vi "Process.vi"(8 "error in":errorcluster, 11 "Log.Litho":refnum<class "Log.Litho.lvclass">) -> (0 "error out":errorcluster, 3 "Log.Litho out":refnum<class "Log.Litho.lvclass">)   [LabVIEW 2019, in "Log.Litho.lvclass"]
doc: "---------------------------------------------------------------\nJKI State Machine Objects™\nhttp://jki.net/state-machine-objects/\nCopyright (C) 2005-2015, JKI <info@jki.net>\nALL RIGHTS RESERVED"
uses:
  Log.Litho.lvclass
  C:/Program Files (x86)/National Instruments/LabVIEW 2019/vi.lib/JKI/JKI SMO/SMO/SMO.lvclass
  <vilib>/JKI/JKI SMO/SMO/Typedefs/Parent Call--Enum.ctl
  <vilib>/JKI/JKI SMO/SMO/SMO.lvclass/SMO.ctl
  Log.Litho.lvclass/Log.Litho.ctl
  <vilib>/JKI/JKI SMO/SMO/Private/ReftoDVR--SMO.vi
  <vilib>/JKI/JKI SMO/SMO/SMO.lvclass
panel:
  # "For instructions on how to use the JKI State Machine Objects, examples and video tutorials, visit:\nhttp://jki.net/state-machine-objects/\n\nJKI State Machine Objects™\nhttp://jki.net/state-machine-objects/\nCopyright (C) 2005-2015, JKI <info@jki.net>\nALL RIGHTS RESERVED"
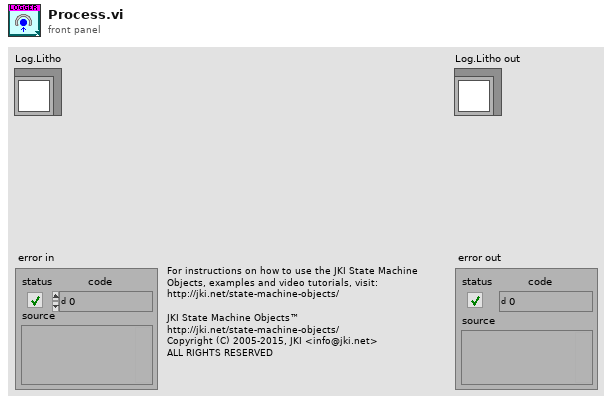
[diagram p1: front panel]
types:
  T1 = typedef "SMO.lvclass/Parent Call--Enum.ctl" = enum16{"Allows parent to run", "Does not request parent to run"}
  T2 = enum32{"invalid app kind", "Development System", "Run Time System", "Student Edition", "Embedded LabVIEW", "Evaluation", "Custom"}
  T3 = enum32{"Invalid", "Standard", "Closed", "Hidden", "Minimized", "Maximized"}
  T4 = enum32{"Bad", "Idle", "Run top level", "Running"}
  T5 = enum16{"open", "replace", "create", "open or create", "replace or create", "replace or create with confirmation"}
  T6 = typedef "Log.Litho.lvclass/PrivateEvents--Log.Litho.Activity.ctl" = string
  T7 = cluster{"Core":cluster{"Current VI Reference":refnum<vi>, "Close Panel on Exit?":bool, "error":errorcluster}, "Self Reference":refnum<class "Log.Litho.lvclass">, "Activity":string, "Path":path, "Active Log":string, "File Refnum":refnum<file>}
  T8 = cluster{"Current VI Reference":refnum<vi>, "Close Panel on Exit?":bool, "error":errorcluster}
  T9 = typedef "SMO.lvclass/Protected Events.ctl" = cluster{"StopProcesses":refnum<user-event>, "AbortProcesses":refnum<user-event>, "Config Changed":refnum<user-event>, "Dependency":refnum<user-event>}
  T10 = typedef "Log.Litho.lvclass/PrivateEvents--Cluster.ctl" = cluster{"Activity":refnum<user-event>}
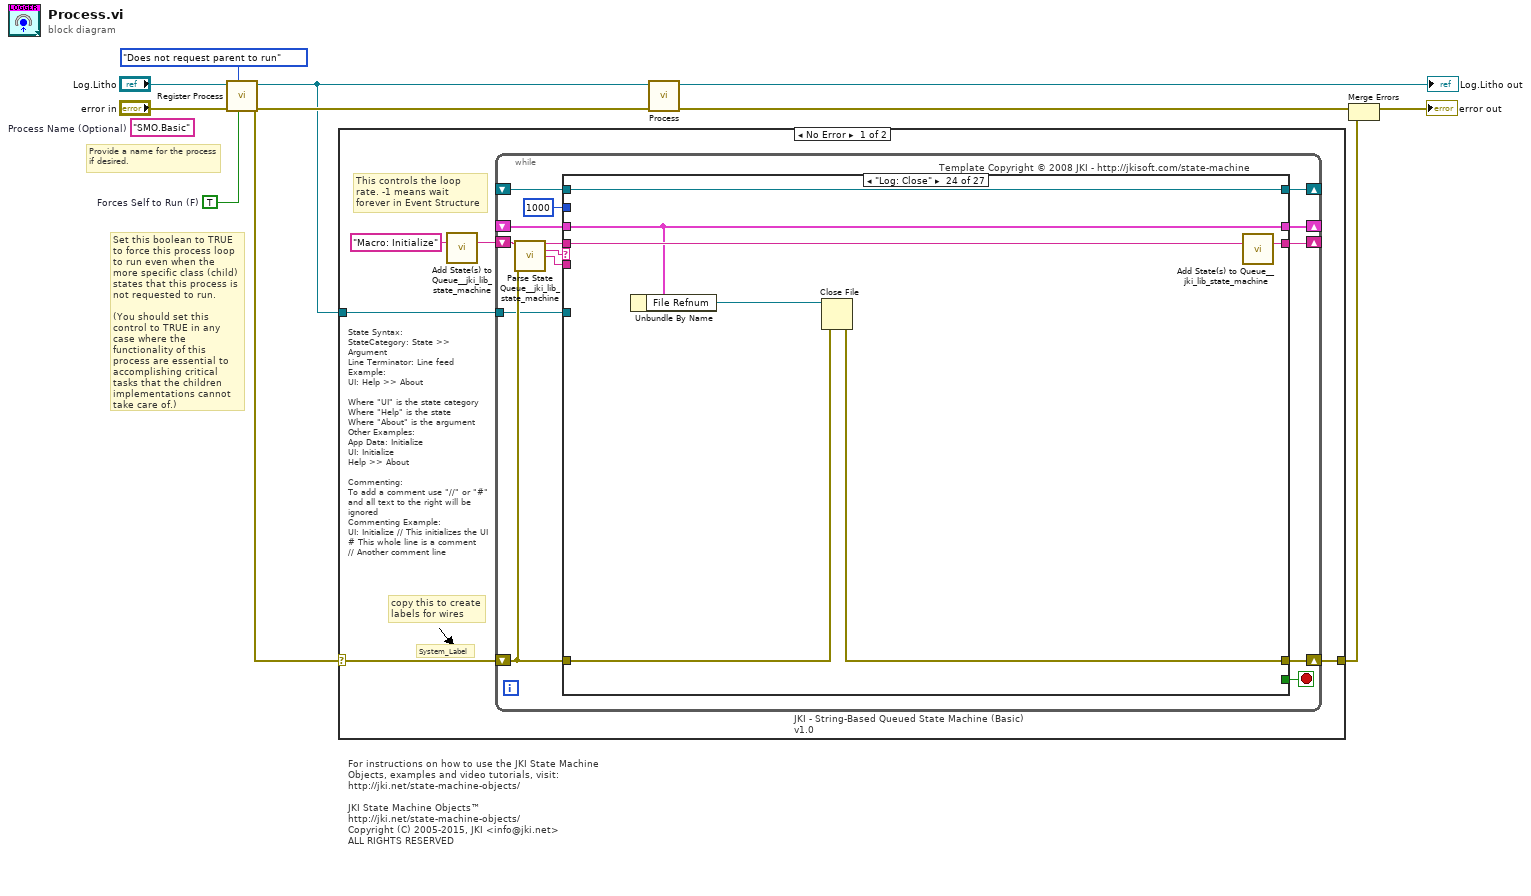
[diagram p0: block diagram]
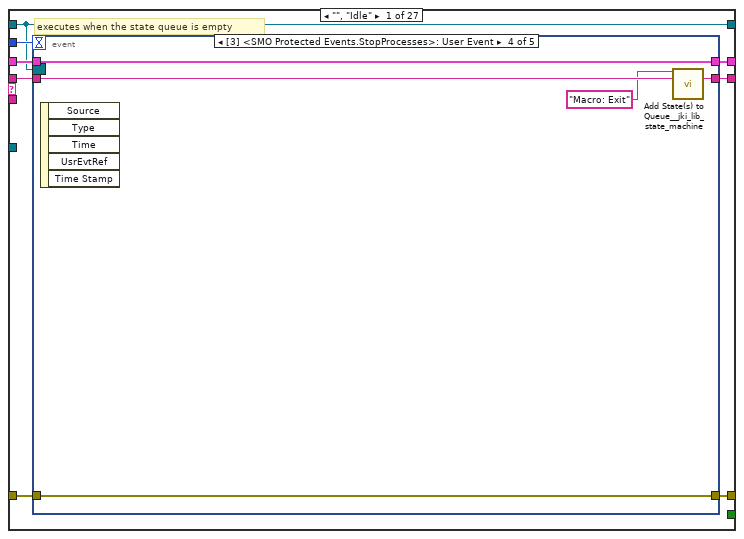
[diagram p2: hidden frame]
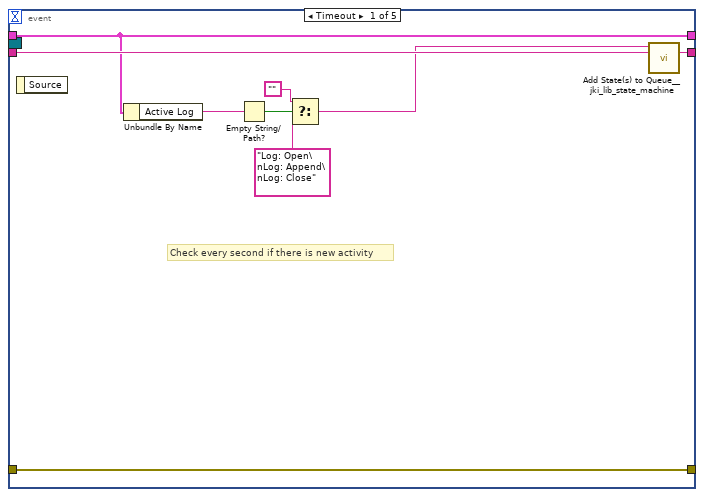
[diagram p3: hidden frame]
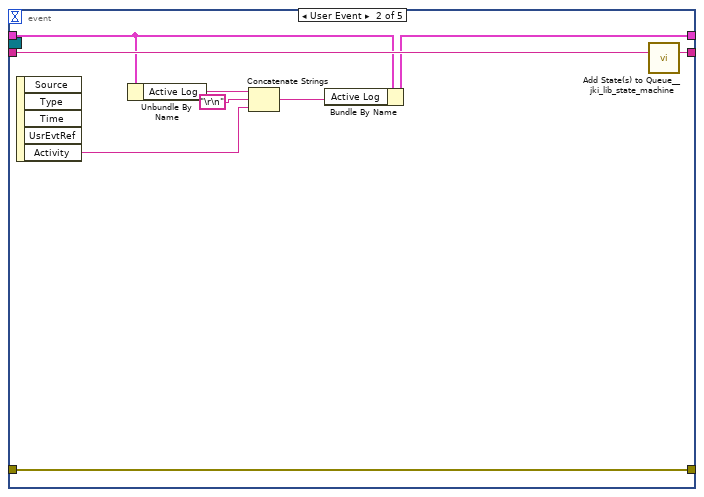
[diagram p4: hidden frame]
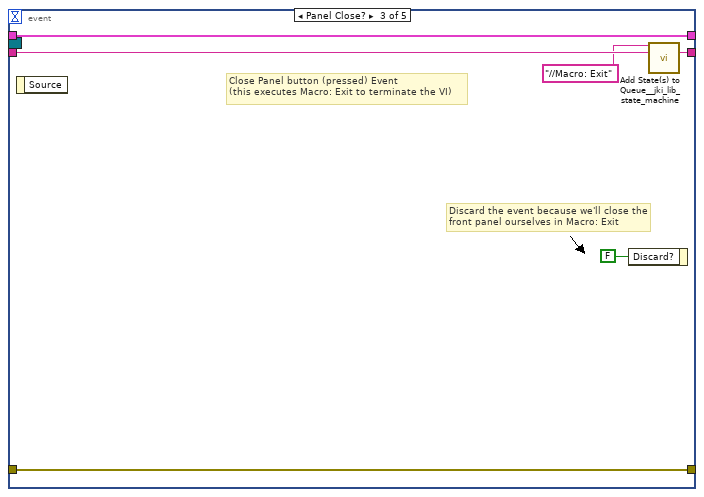
[diagram p5: hidden frame]
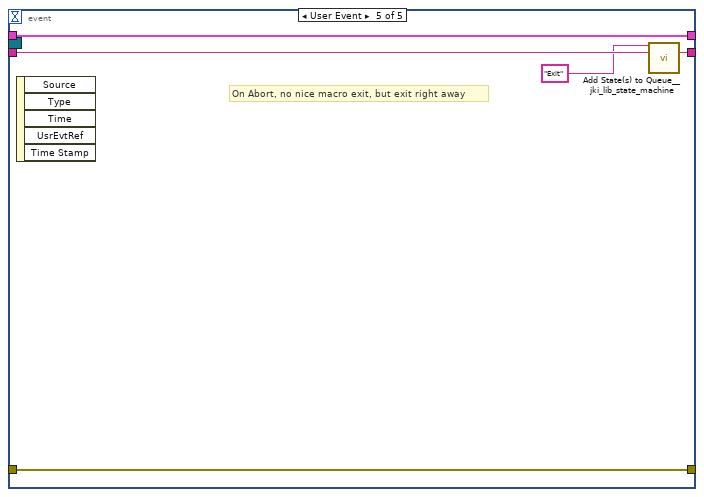
[diagram p6: hidden frame]
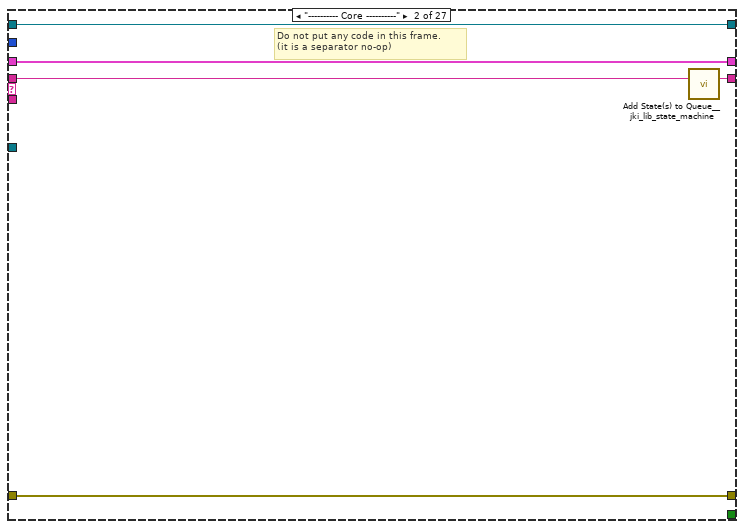
[diagram p7: hidden frame]
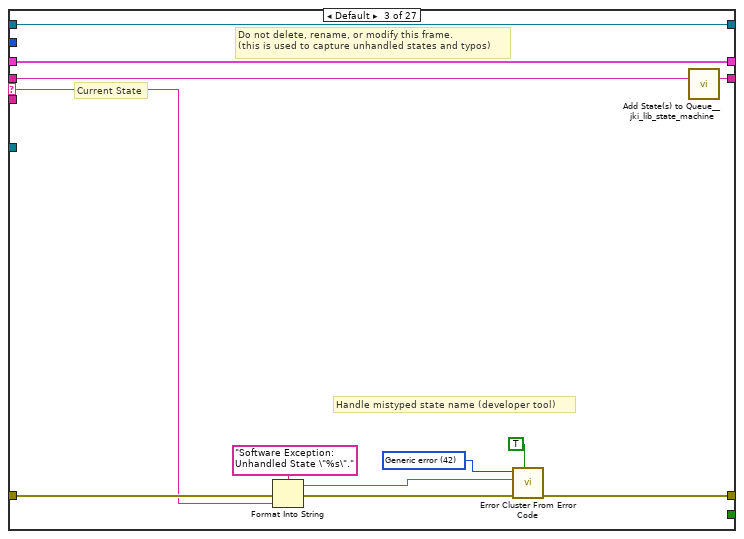
[diagram p8: hidden frame]
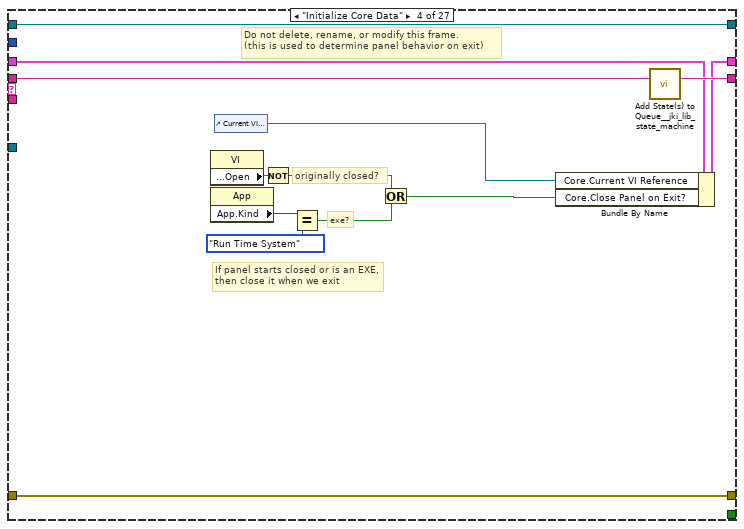
[diagram p9: hidden frame]
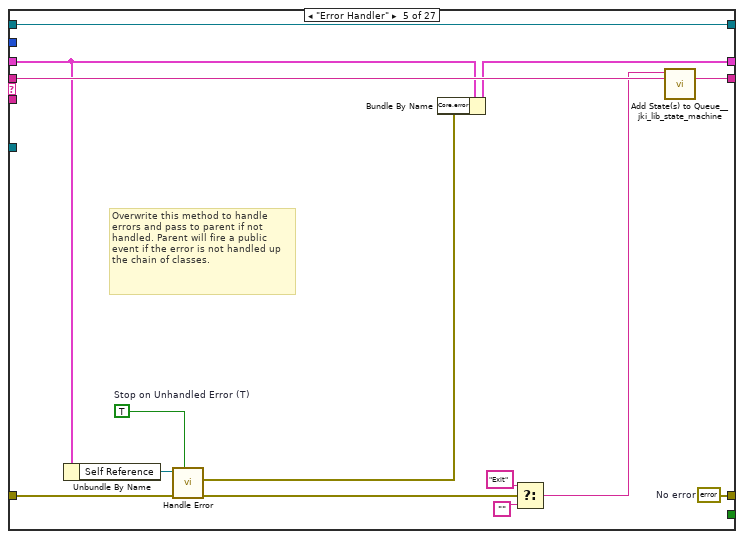
[diagram p10: hidden frame]
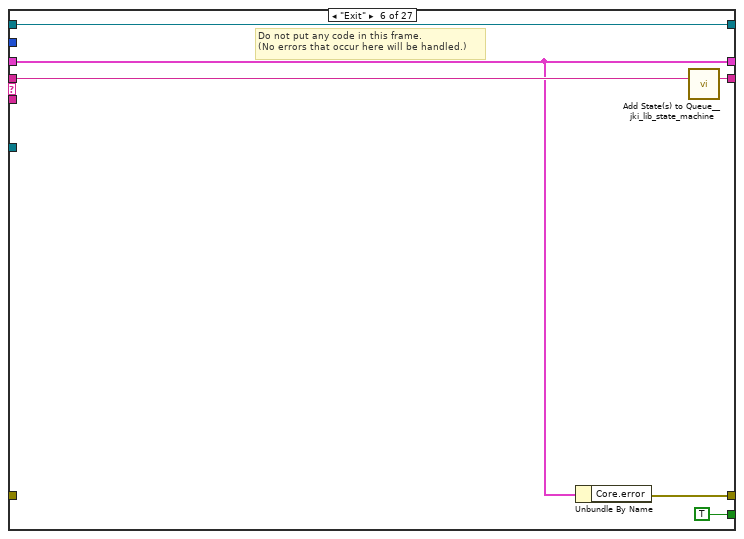
[diagram p11: hidden frame]
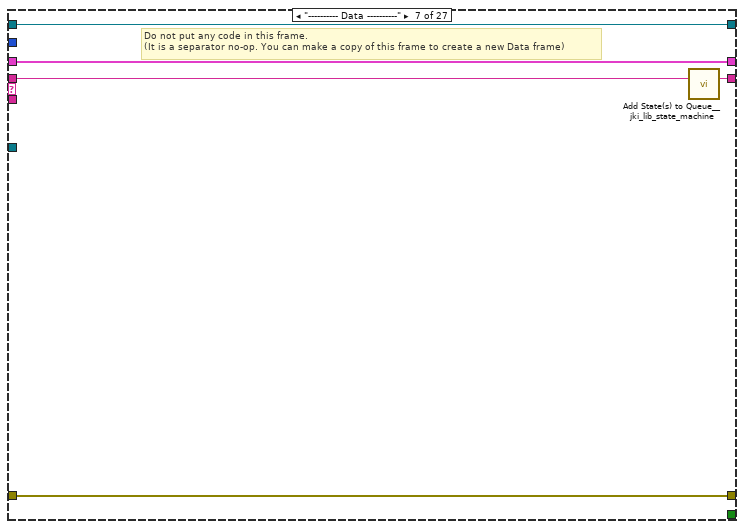
[diagram p12: hidden frame]
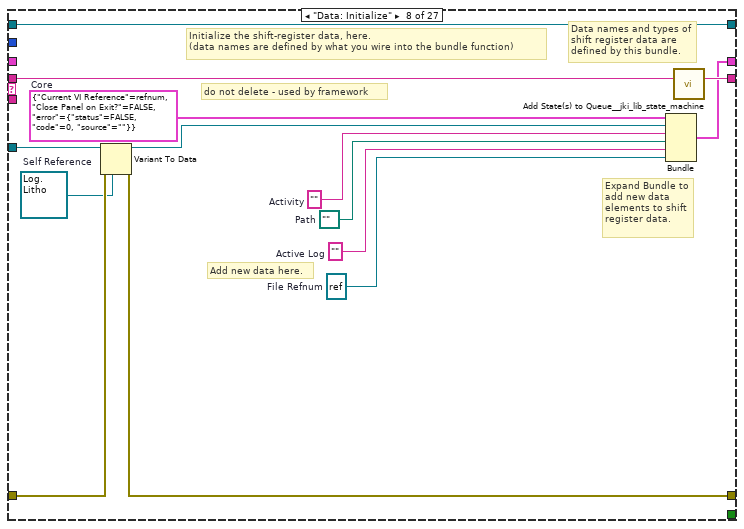
[diagram p13: hidden frame]
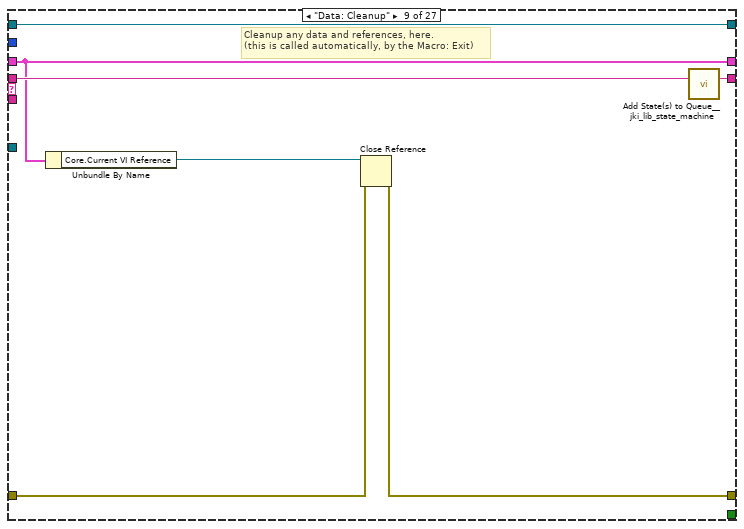
[diagram p14: hidden frame]
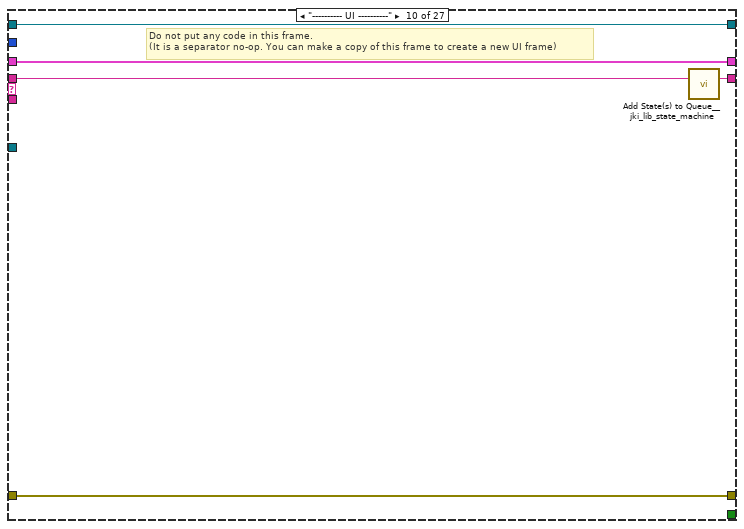
[diagram p15: hidden frame]
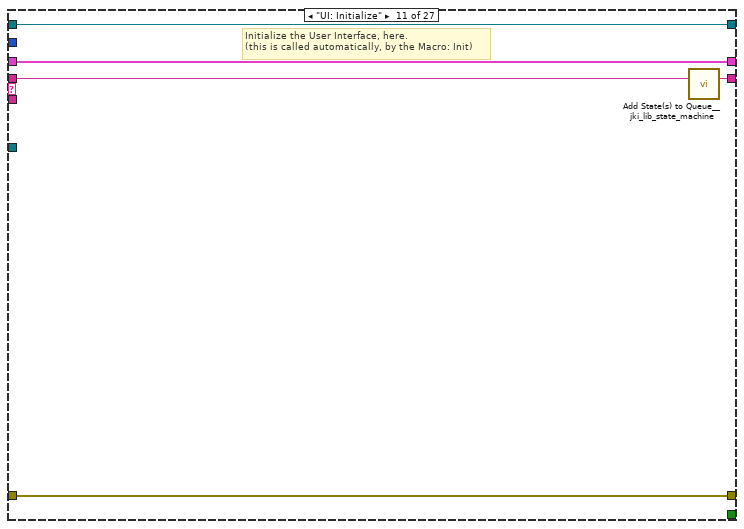
[diagram p16: hidden frame]
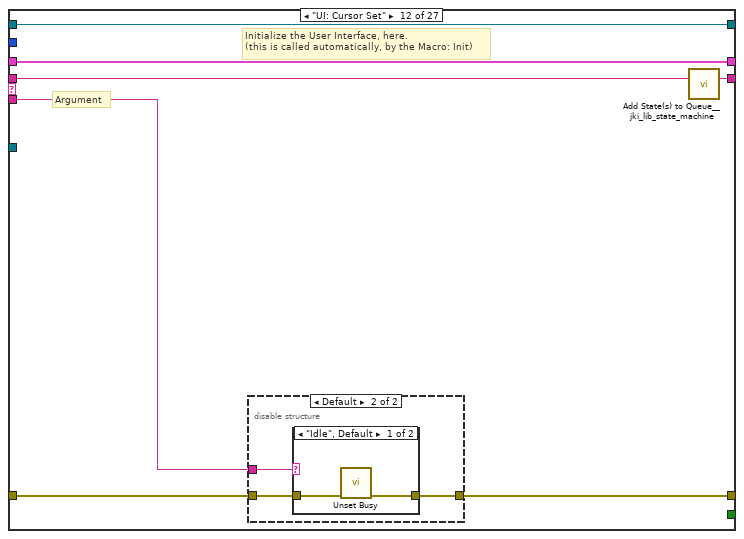
[diagram p17: hidden frame]
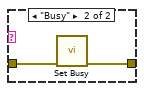
[diagram p19: hidden frame]
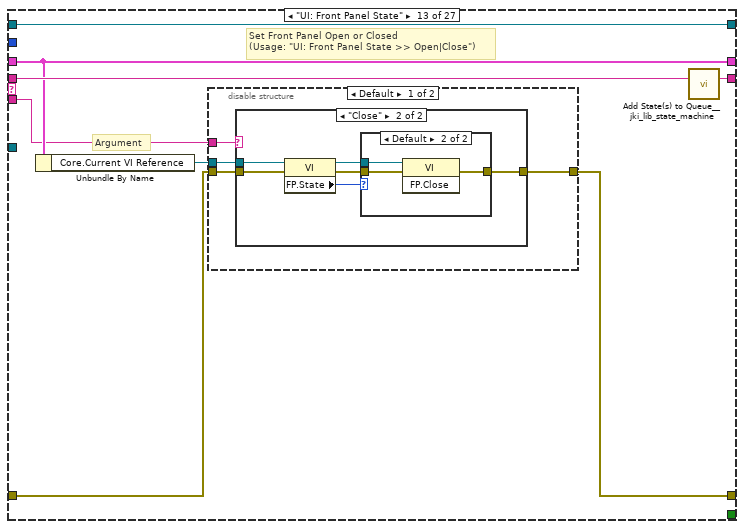
[diagram p20: hidden frame]
diagram:
  w1 = TRUE  # Forces Self to Run (F)
  (unwired) "SMO.Basic"  # Process Name (Optional)
  # "Provide a name for the process\nif desired."
  # "Set this boolean to TRUE to force this process loop to run even when the more specific class (child) states that this process is not requested to run.\n\n(You should set this control to TRUE in any case where the functionality of this process are essential to accomplishing critical tasks that the children implementations cannot take care of.)"
  # "For instructions on how to use the JKI State Machine Objects, examples and video tutorials, visit:\nhttp://jki.net/state-machine-objects/\n\nJKI State Machine Objects™\nhttp://jki.net/state-machine-objects/\nCopyright (C) 2005-2015, JKI <info@jki.net>\nALL RIGHTS RESERVED"
  n1 = call <vilib>:"Register Process.vi"("Forces Self to Run (F)"=w1, "Parent Call"=Parent_Call--Enum."Does not request parent to run", "error in (no error)"="error in", "SMO"="Log.Litho") -> ("error out"=w7:errorcluster, "SMO out"=w6:refnum<class "Log.Litho.lvclass">)  [unwired: 6 in]
  n2 = case shown="No Error" w7 {
    selector: w7 -> [w12 w342]
    tunnel: w6 -> [w13 _]
    tunnel: [w11 w342] -> w3
    frame No Error {
      # "State Syntax:\nStateCategory: State >> Argument\nLine Terminator: Line feed\nExample:\nUI: Help >> About\n\nWhere \"UI\" is the state category\nWhere \"Help\" is the state\nWhere \"About\" is the argument\nOther Examples:\nApp Data: Initialize\nUI: Initialize\nHelp >> About\n\nCommenting:\nTo add a comment use \"//\" or \"#\" and all text to the right will be ignored\nCommenting Example:\nUI: Initialize // This initializes the UI\n# This whole line is a comment\n// Another comment line"
      # "copy this to create labels for wires"
      # "This controls the loop rate. -1 means wait forever in Event Structure"
      # "System_Label"
      n3 = call <vilib>:"Add State(s) to Queue__jki_lib_state_machine.vi"("State(s) in (\"\")"="Macro: Initialize") -> ("States Out"=w15:string)  [unwired: 14 in]
      n4 = while "JKI - String-Based Queued State Machine (Basic) v1.0" {
        shift-right: [w22] -> _
        shift-left: _ -> [w21]
        shift-right: [w25] -> w11
        shift-left: w12 -> [w19]
        shift-right: [w24] -> _
        shift-left: w15 -> [w26]
        tunnel: w13 -> [w18]
        shift-right: [w17] -> _
        shift-left: _ -> [w16]
        stop <- w23 stop-if-true
        # "Template Copyright © 2008 JKI - http://jkisoft.com/state-machine"
        n5 = call <vilib>:"Parse State Queue__jki_lib_state_machine.vi"("State Queue"=w26, "Error In (no error)"=w19) -> ("Remaining States"=w28:string, "Current State"=w29:string, "Arguments"=w27:string)  [unwired: 11 in]
        n6 = case shown="\"Log: Close\"" w29 {
          selector: w29 -> [_ _ w78 _ _ _ _ _ _ _ _ _ _ _ _ _ _ _ _ _ _ _ _ _ _ _ _]
          tunnel: w28 -> [w37 w76 w82 w101 w115 w121 w126 w140 w147 w152 w157 w164 w180 w212 w226 w240 w245 w256 w261 w273 w279 w284 w300 w307 w317 w333 w341]
          tunnel: w27 -> [_ _ _ _ _ _ _ _ _ _ _ w158 w174 _ _ _ _ _ _ _ _ _ _ _ _ _ _]
          tunnel: w21 -> [w35 w73 w80 w92 w109 w117 w123 _ w142 w149 w155 w162 w176 w209 w222 w231 w242 w253 w258 w271 w277 w282 w288 w304 w308 w320 w334]
          tunnel: [w34 w74 w84 w98 w110 w116 w124 w135 w143 w150 w154 w159 w177 w210 w224 w238 w243 w247 w259 w267 w275 w280 w291 w302 w312 w323 w337] -> w25
          tunnel: w19 -> [w33 w74 w83 w98 w111 _ w124 w136 w144 w150 w154 w160 w178 w210 w224 w238 w243 w248 w259 w268 w275 w280 w290 w301 w311 w322 w338]
          tunnel: [w36 w75 w81 w100 w114 w120 w125 w139 w146 w151 w156 w163 w179 w211 w225 w239 w244 w255 w260 w272 w278 w283 w299 w306 w316 w332 w340] -> w24
          tunnel: [_ _ _ _ _ TRUE _ _ _ _ _ _ _ _ _ _ _ _ _ _ _ _ _ _ _ _ _] -> w23
          tunnel: [w32 w73 w80 w99 w108 w117 w123 w138 w142 w149 w155 w162 w176 w209 w222 w231 w242 w253 w258 w271 w277 w282 w289 w304 w309 w321 w335] -> w22
          tunnel: 1000 ("Timeout") -> [w31 _ _ _ _ _ _ _ _ _ _ _ _ _ _ _ _ _ _ _ _ _ _ _ _ _ _]
          tunnel: w18 -> [_ _ _ _ _ _ _ w133 _ _ _ _ _ _ _ _ _ _ _ _ _ _ _ _ _ _ _]
          tunnel: [w30 w72 w77 w89 w113 w118 w122 w131 w141 w148 w153 w161 w173 w208 w223 w232 w241 w254 w257 w270 w276 w281 w298 w305 w315 w331 w339] -> w17
          tunnel: w16 -> [w30 w72 w77 w89 w113 w118 w122 w131 w141 w148 w153 w161 w173 w208 w223 w232 w241 w254 w257 _ w276 w281 w298 w305 w315 w331 w339]
          frame "", "Idle" {
            # "executes when the state queue is empty"
            n7 = event shown="[3] <SMO Protected Events.StopProcesses>: User Event" {
              selector: w30 -> [_ _ _ _ _]
              dyn-events: _ -> [_ _ _ _ _]
              timeout: w31 -> [_ _ _ _ _]
              tunnel: w37 -> [w46 w55 w61 w66 w71]
              tunnel: [w45 w54 w60 w65 w70] -> w36
              tunnel: w35 -> [w43 w49 w58 w63 w68]
              tunnel: [w44 w53 w59 w64 w69] -> w34
              tunnel: w33 -> [w44 w53 w59 w64 w69]
              tunnel: [w43 w50 w58 w63 w68] -> w32
              event Timeout {
                # "Check every second if there is new activity"
                n8 = event-data() -> ()  [unwired: 1 in, 1 out]
                n9 = Unbundle By Name(w43) -> ("Active Log"=w42:string)
                n10 = Empty String/Path?(string/path=w42) -> (empty?=w41:bool)
                n11 = Select(t="", s=w41, f="Log: Open\nLog: Append\nLog: Close") -> (s? t:f=w38:string)
                n12 = call <vilib>:"Add State(s) to Queue__jki_lib_state_machine.vi"("State(s) in Front (\"\")"=w38, "State(s) in (\"\")"=w46) -> ("States Out"=w45:string)  [unwired: 13 in]
              }
              event User Event {
                n13 = event-data() -> ("Activity"=w48:T6)  [unwired: 1 in, 4 out]
                n14 = Unbundle By Name(w49) -> ("Active Log"=w52:string)
                n15 = Concatenate Strings(w52, "\r\n", w48) -> (w47:string)
                n16 = Bundle By Name(cluster=w49, "Active Log"=w47) -> (w50:T7)
                n17 = call <vilib>:"Add State(s) to Queue__jki_lib_state_machine.vi"("State(s) in (\"\")"=w55) -> ("States Out"=w54:string)  [unwired: 14 in]
              }
              event Panel Close? {
                # "Discard the event because we'll close the front panel ourselves in Macro: Exit"
                # "Close Panel button (pressed) Event\n(this executes Macro: Exit to terminate the VI)"
                n18 = event-data() -> ()  [unwired: 1 in, 1 out]
                n19 = event-data("Discard?"=FALSE) -> ()  [unwired: 1 in, 1 out]
                n20 = call <vilib>:"Add State(s) to Queue__jki_lib_state_machine.vi"("State(s) in Front (\"\")"="//Macro: Exit", "State(s) in (\"\")"=w61) -> ("States Out"=w60:string)  [unwired: 13 in]
              }
              event User Event {
                n21 = event-data() -> ()  [unwired: 1 in, 5 out]
                n22 = call <vilib>:"Add State(s) to Queue__jki_lib_state_machine.vi"("State(s) in Front (\"\")"="Macro: Exit", "State(s) in (\"\")"=w66) -> ("States Out"=w65:string)  [unwired: 13 in]
              }
              event User Event {
                # "On Abort, no nice macro exit, but exit right away"
                n23 = event-data() -> ()  [unwired: 1 in, 5 out]
                n24 = call <vilib>:"Add State(s) to Queue__jki_lib_state_machine.vi"("State(s) in Front (\"\")"="Exit", "State(s) in (\"\")"=w71) -> ("States Out"=w70:string)  [unwired: 13 in]
              }
            }
          }
          frame "---------- Core ----------" {
            # "Do not put any code in this frame.\n(it is a separator no-op)"
            n25 = call <vilib>:"Add State(s) to Queue__jki_lib_state_machine.vi"("State(s) in (\"\")"=w76) -> ("States Out"=w75:string)  [unwired: 14 in]
          }
          frame Default {
            w87 = 42 items=["No error", "Argument error", "Memory is full", "Out of zone", "End of file", "File already open", "Generic file I/O error", "File not found", "File permission error", "Disk is full", "Duplicate path", "Too many files open", "System feature not enabled", "Resource file not found", "Cannot add resource", "Resource not found", "Image not found", "Image memory error", "Pen does not exist", "Config type invalid", "Config token not found", "Config parse error", "Config memory error", "Bad external code format", "Bad external code offset", "External code not present", "Null window", "Destroy window error", "Null menu", "Print aborted", "Bad print record", "Print driver error", "Windows error during printing", "Memory error during printing", "Print dialog error", "Generic print error", "Invalid device refnum", "Device not found", "Device parameter error", "Device unit error", "Cannot open device", "Device call aborted", "Generic error", "Cancelled by user", "Object ID too low", "Object ID too high", "Object not in heap", "Unknown heap", "Unknown object (invalid DefProc)", "Unknown object (DefProc not in table)", "Message out of range", "Invalid (null) method", "Unknown message", "Manager call not supported", "Bad address", "Network operation in progress", "Network operation timed out", "Connection is busy", "Network attribute not supported", "Network error", "Address in use", "System out of memory", "Connection aborted", "Connection refused", "Not connected", "Already connected", "Connection closed", "Initialization error (interapplication manager)", "Bad occurrence", "Wait on unbound occurrence handler", "Occurrence queue overflow", "Datalog type conflict", "Unused", "Unrecognized type (interapplication manager)", "Memory corrupt", "Failed to make temporary DLL", "Old CIN version", "Drag socket not found", "Failed to load drop-object", "Failed to register OLE object", "Failed to release OLE object", "Format specifier type mismatch", "Unknown format specifier", "Too few format specifiers", "Too many format specifiers", "Scan failed", "Newer CIN version", "Error converting to variant", "Runtime menu error", "Password tampered", "Variant attribute not found", "Incompatible variant data type", "Event data is not available", "Event Store is not present", "Occurrence is not found", "Event Queue is not created", "Event info is not available", "Refnum passed is NULL", "Error retrieving Class GUID", "Error retrieving CoClass GUID", "Error retrieving TypeLib GUID.", "Bad built application magic bytes.", "Specific driver is different from the specific driver associated with the Logical Name.", "There is no session opened to the class driver.", "Max Error", "MAX - Error with config objects", "MAX - Error loading configuration", "MAX - Group not supported"]
            # "Current State"
            # "Do not delete, rename, or modify this frame.\n(this is used to capture unhandled states and typos)"
            # "Handle mistyped state name (developer tool)"
            n26 = Format Into String(format string="Software Exception: Unhandled State \"%s\"." ("message"), error in=w83, w78) -> (resulting string=w86:string, error out=w85:errorcluster)  [unwired: 1 in]
            n27 = call <vilib>:"Error Cluster From Error Code.vi"("show call chain? (False)"=TRUE, "error in (no error)"=w85, "error message (\"\")"=w86, "error code (0)"=w87) -> ("error out"=w84:errorcluster)  [unwired: 5 in]
            n28 = call <vilib>:"Add State(s) to Queue__jki_lib_state_machine.vi"("State(s) in (\"\")"=w82) -> ("States Out"=w81:string)  [unwired: 14 in]
          }
          frame "Initialize Core Data" {
            # "Do not delete, rename, or modify this frame.\n(this is used to determine panel behavior on exit)"
            # "originally closed?"
            # "exe?"
            # "If panel starts closed or is an EXE, then close it when we exit"
            n29 = property class="VI"() -> ("Front Panel.Open"=w97:bool)  [unwired: 2 in, 2 out]
            n30 = property class="App"() -> ("App.Kind"=w96:T2)  [unwired: 2 in, 2 out]
            n31 = control-ref of="Current VI Reference"() -> (w90:refnum<vi>)
            n32 = Not(x=w97) -> (.not. x?=w94:bool)
            n33 = Equal?(x=w96, y=T2."Run Time System" ("Application:Kind")) -> (x = y?=w93:bool)
            n34 = Or(x=w94, y=w93) -> (x .or. y?=w91:bool)
            n35 = Bundle By Name(cluster=w92, "Core.Current VI Reference"=w90, "Core.Close Panel on Exit?"=w91) -> (w99:T7)
            n36 = call <vilib>:"Add State(s) to Queue__jki_lib_state_machine.vi"("State(s) in (\"\")"=w101) -> ("States Out"=w100:string)  [unwired: 14 in]
          }
          frame "Error Handler" {
            w102 = TRUE  # Stop on Unhandled Error (T)
            w110 = errorcluster {"status"=FALSE, "code"=0, "source"=""}  # No error
            # "Overwrite this method to handle errors and pass to parent if not handled. Parent will fire a public event if the error is not handled up the chain of classes."
            n37 = Unbundle By Name(w109) -> ("Self Reference"=w112:refnum<class "Log.Litho.lvclass">)
            n38 = call-dynamic "Handle Error.vi"("Stop on Unhandled Error (T)"=w102, "error in"=w111, "SMO"=w112) -> ("handling error"=w103:errorcluster, "Unhandled error"=w106:errorcluster)  [unwired: 6 in, 1 out]
            n39 = Bundle By Name(cluster=w109, "Core.error"=w106) -> (w108:T7)
            n40 = Select(t="Exit", s=w103, f="") -> (s? t:f=w107:string)
            n41 = call <vilib>:"Add State(s) to Queue__jki_lib_state_machine.vi"("State(s) in Front (\"\")"=w107, "State(s) in (\"\")"=w115) -> ("States Out"=w114:string)  [unwired: 13 in]
          }
          frame "Exit" {
            # "Do not put any code in this frame.\n(No errors that occur here will be handled.)"
            n42 = Unbundle By Name(w117) -> ("Core.error"=w116:errorcluster)
            n43 = call <vilib>:"Add State(s) to Queue__jki_lib_state_machine.vi"("State(s) in (\"\")"=w121) -> ("States Out"=w120:string)  [unwired: 14 in]
          }
          frame "---------- Data ----------" {
            # "Do not put any code in this frame.\n(It is a separator no-op. You can make a copy of this frame to create a new Data frame)"
            n44 = call <vilib>:"Add State(s) to Queue__jki_lib_state_machine.vi"("State(s) in (\"\")"=w126) -> ("States Out"=w125:string)  [unwired: 14 in]
          }
          frame "Data: Initialize" {
            w127 = refnum<file> refnum  # File Refnum
            w128 = ""  # Active Log
            w129 = path ""  # Path
            w130 = T8 {"Current VI Reference"=refnum, "Close Panel on Exit?"=FALSE, "error"={"status"=FALSE, "code"=0, "source"=""}}  # Core
            w134 = refnum<class "Log.Litho.lvclass"> refnum  # Self Reference
            w137 = ""  # Activity
            # "do not delete - used by framework"
            # "Expand Bundle to add new data elements to shift register data."
            # "Add new data here."
            # "Data names and types of shift register data are defined by this bundle."
            # "Initialize the shift-register data, here.\n(data names are defined by what you wire into the bundle function)"
            n45 = Variant To Data(error in=w136, type=w134, Variant=w133) -> (data=w132:refnum<class "Log.Litho.lvclass">, error out=w135:errorcluster)
            n46 = Bundle("Core"=w130, "Self Reference"=w132, "Activity"=w137, "Path"=w129, "Active Log"=w128, "File Refnum"=w127) -> (w138:T7)  [unwired: 1 in]
            n47 = call <vilib>:"Add State(s) to Queue__jki_lib_state_machine.vi"("State(s) in (\"\")"=w140) -> ("States Out"=w139:string)  [unwired: 14 in]
          }
          frame "Data: Cleanup" {
            # "Cleanup any data and references, here.\n(this is called automatically, by the Macro: Exit)"
            n48 = Unbundle By Name(w142) -> ("Core.Current VI Reference"=w145:refnum<vi>)
            n49 = Close Reference(reference=w145, error in (no error)=w144) -> (error out=w143:errorcluster)
            n50 = call <vilib>:"Add State(s) to Queue__jki_lib_state_machine.vi"("State(s) in (\"\")"=w147) -> ("States Out"=w146:string)  [unwired: 14 in]
          }
          frame "---------- UI ----------" {
            # "Do not put any code in this frame.\n(It is a separator no-op. You can make a copy of this frame to create a new UI frame)"
            n51 = call <vilib>:"Add State(s) to Queue__jki_lib_state_machine.vi"("State(s) in (\"\")"=w152) -> ("States Out"=w151:string)  [unwired: 14 in]
          }
          frame "UI: Initialize" {
            # "Initialize the User Interface, here.\n(this is called automatically, by the Macro: Init)"
            n52 = call <vilib>:"Add State(s) to Queue__jki_lib_state_machine.vi"("State(s) in (\"\")"=w157) -> ("States Out"=w156:string)  [unwired: 14 in]
          }
          frame "UI: Cursor Set" {
            # "Argument"
            # "Initialize the User Interface, here.\n(this is called automatically, by the Macro: Init)"
            n53 = disable-structure shown="Default" {
              disable-tunnel: w160 -> [w165 w168]
              disable-tunnel: [w165 w167] -> w159
              disable-tunnel: w158 -> [_ w166]
              frame condition #0 {
              }
              frame condition #1 (active) {
                n54 = case shown="\"Idle\", Default" w166 {
                  tunnel: w168 -> [w170 w172]
                  tunnel: [w169 w171] -> w167
                  frame "Idle", Default {
                    n55 = call <vilib>:"Unset Busy.vi"("error in (no error)"=w170) -> ("error out"=w169:errorcluster)  [unwired: 10 in]
                  }
                  frame "Busy" {
                    n56 = call <vilib>:"Set Busy.vi"("error in (no error)"=w172) -> ("error out"=w171:errorcluster)  [unwired: 9 in, 1 out]
                  }
                }
              }
            }
            n57 = call <vilib>:"Add State(s) to Queue__jki_lib_state_machine.vi"("State(s) in (\"\")"=w164) -> ("States Out"=w163:string)  [unwired: 14 in]
          }
          frame "UI: Front Panel State" {
            # "Argument"
            # "Set Front Panel Open or Closed\n(Usage: \"UI: Front Panel State >> Open|Close\")"
            n58 = Unbundle By Name(w176) -> ("Core.Current VI Reference"=w175:refnum<vi>)
            n59 = disable-structure shown="Default" {
              disable-tunnel: w178 -> [w184 w207]
              disable-tunnel: [w183 w207] -> w177
              disable-tunnel: w175 -> [w182 _]
              disable-tunnel: w174 -> [w181 _]
              frame condition #0 (active) {
                n60 = case shown="\"Close\"" w181 {
                  tunnel: w184 -> [w188 w201]
                  tunnel: [w190 w202] -> w183
                  tunnel: w182 -> [w189 w199]
                  frame "Open", Default {
                    n61 = property class="VI"(reference=w189, error in=w188) -> (reference out=w186:refnum<vi>, error out=w187:errorcluster, "FP.State"=w185:T3)
                    n62 = case shown="\"Closed\"" w185 {
                      tunnel: [w193 w196] -> w190
                      tunnel: w187 -> [w192 w196]
                      tunnel: w186 -> [w191 _]
                      frame "Closed" {
                        n63 = invoke class="VI" method="FP.Open"(reference=w191, error in=w192, "Activate"=TRUE, "State"=T3."Standard") -> (error out=w193:errorcluster)  [unwired: 1 in, 4 out]
                      }
                      frame Default {
                      }
                    }
                  }
                  frame "Close" {
                    n64 = property class="VI"(reference=w199, error in=w201) -> (reference out=w198:refnum<vi>, error out=w200:errorcluster, "FP.State"=w197:T3)
                    n65 = case shown="Default" w197 {
                      tunnel: [w203 w206] -> w202
                      tunnel: w200 -> [w203 w205]
                      tunnel: w198 -> [_ w204]
                      frame "Invalid", "Closed" {
                      }
                      frame Default {
                        n66 = invoke class="VI" method="FP.Close"(reference=w204, error in=w205) -> (error out=w206:errorcluster)  [unwired: 1 in, 2 out]
                      }
                    }
                  }
                }
              }
              frame condition #1 {
              }
            }
            n67 = call <vilib>:"Add State(s) to Queue__jki_lib_state_machine.vi"("State(s) in (\"\")"=w180) -> ("States Out"=w179:string)  [unwired: 14 in]
          }
          frame "---------- Macro ----------" {
            # "Do not put any code in this frame.\n(It is a separator no-op. You can make a copy of this frame to create a new Macro frame)"
            n68 = call <vilib>:"Add State(s) to Queue__jki_lib_state_machine.vi"("State(s) in (\"\")"=w212) -> ("States Out"=w211:string)  [unwired: 14 in]
          }
          frame "Macro: Initialize" {
            w217 = "//UI: Initialize\n//UI: Front Panel State >> Open"  # //UI: Initialize //UI: Front Panel State >> Open
            w213 = "Process: Sync"
            # "Initialization Macro\n(This is called once, when the VI starts)"
            n69 = control-ref of="This VI"() -> (w215:refnum<vi>)
            n70 = property class="VI"(reference=w215) -> ("Exec.State"=w214:T4)  [unwired: 1 in, 2 out]
            n71 = Equal?(x=w214, y=T4."Run top level") -> (x = y?=w220:bool)
            n72 = Select(t=w213, s=w220, f="") -> ()  [unwired: 1 out]
            n73 = call <vilib>:"Add State(s) to Queue__jki_lib_state_machine.vi"("State(s) in Front (\"\")"="Data: Initialize\nInitialize Core Data\nEvents: Register\nLog: Path\nLog: Log Offline", "State(s) in (\"\")"=w213, "State(s) at Back (\"\")"=w217) -> ("States Out"=w216:string)  [unwired: 12 in]
            n74 = call <vilib>:"Add State(s) to Queue__jki_lib_state_machine.vi"("State(s) in Front (\"\")"=w216, "State(s) in (\"\")"=w226) -> ("States Out"=w225:string)  [unwired: 13 in]
          }
          frame "Macro: Exit" {
            # "Exit Macro\n(This is called once, when the VI exits)"
            n75 = Unbundle By Name(w231) -> ("Core.Close Panel on Exit?"=w237:bool)
            n76 = Select(t="UI: Front Panel State >> Close", s=w237, f="") -> (s? t:f=w234:string)
            n77 = call <vilib>:"Add State(s) to Queue__jki_lib_state_machine.vi"("State(s) in Front (\"\")"="Log: Open\nLog: Append\nLog: Close\nData: Cleanup\nEvents: Unregister", "State(s) in (\"\")"="Process: Sync", "State(s) at Back (\"\")"="Exit") -> ("States Out"=w228:string)  [unwired: 12 in]
            n78 = call <vilib>:"Add State(s) to Queue__jki_lib_state_machine.vi"("State(s) in (\"\")"=w234, "State(s) at Back (\"\")"=w228) -> ("States Out"=w233:string)  [unwired: 13 in]
            n79 = call <vilib>:"Add State(s) to Queue__jki_lib_state_machine.vi"("State(s) in Front (\"\")"=w233, "State(s) in (\"\")"=w240) -> ("States Out"=w239:string)  [unwired: 13 in]
          }
          frame "---------- Process ----------" {
            # "Template Separator\n(You can make a copy of, or modify, this frame)"
            n80 = call <vilib>:"Add State(s) to Queue__jki_lib_state_machine.vi"("State(s) in (\"\")"=w245) -> ("States Out"=w244:string)  [unwired: 14 in]
          }
          frame "Process: Sync" {
            n81 = Unbundle By Name(w253) -> ("Self Reference"=w249:refnum<class "Log.Litho.lvclass">)
            n82 = call <vilib>:"WaitOnProcessSync.vi"("error in (no error)"=w248, "SMO"=w249) -> ("error out"=w247:errorcluster, "Don't run?"=w252:bool)  [unwired: 7 in, 1 out]
            n83 = Select(t="Data: Cleanup\nEvents: Unregister\nExit", s=w252, f="") -> (s? t:f=w246:string)
            n84 = call <vilib>:"Add State(s) to Queue__jki_lib_state_machine.vi"("State(s) in Front (\"\")"=w246, "State(s) in (\"\")"=w256) -> ("States Out"=w255:string)  [unwired: 13 in]
          }
          frame "---------- Events ----------" {
            # "Template Separator\n(You can make a copy of, or modify, this frame)"
            n85 = call <vilib>:"Add State(s) to Queue__jki_lib_state_machine.vi"("State(s) in (\"\")"=w261) -> ("States Out"=w260:string)  [unwired: 14 in]
          }
          frame "Events: Register" {
            # "Expand to add\nmore events"
            n86 = Unbundle By Name(w271) -> ("Self Reference"=w264:refnum<class "Log.Litho.lvclass">)
            n87 = call <vilib>:"GetProtectedEvents.vi"("SMO"=w264) -> ("error out"=w265:errorcluster, "SMO Protected Events"=w269:T9)  [unwired: 8 in, 1 out]
            n88 = call "Log.Litho.GetPrivateEvents.vi"("Log.Litho"=w264) -> ("error out"=w262:errorcluster, "Private Events"=w263:T10)  [unwired: 8 in, 1 out]
            n89 = register-events(w269, w263) -> (reference out=w270:refnum<event-registration>, error out=w266:errorcluster)  [unwired: 2 in]
            n90 = Merge Errors(w268, w266, w265, w262) -> (w267:errorcluster)
            n91 = call <vilib>:"Add State(s) to Queue__jki_lib_state_machine.vi"("State(s) in (\"\")"=w273) -> ("States Out"=w272:string)  [unwired: 14 in]
          }
          frame "Events: Unregister" {
            n92 = Unregister For Events(event registration refnum=w276, error in=w275) -> (error out=w274:errorcluster)
            n93 = call <vilib>:"Clear Errors.vi"("error in (no error)"=w274) -> ()  [unwired: 5 in, 2 out]
            n94 = call <vilib>:"Add State(s) to Queue__jki_lib_state_machine.vi"("State(s) in (\"\")"=w279) -> ("States Out"=w278:string)  [unwired: 14 in]
          }
          frame "---------- Log ----------" {
            n95 = call <vilib>:"Add State(s) to Queue__jki_lib_state_machine.vi"("State(s) in (\"\")"=w284) -> ("States Out"=w283:string)  [unwired: 14 in]
          }
          frame "Log: Log Offline" {
            n96 = Unbundle By Name(w288) -> ("Self Reference"=w287:refnum<class "Log.Litho.lvclass">, "Path"=w286:path)
            n97 = Unbundle By Name(w287) -> ("Offline Log"=w295:string)
            n98 = Open/Create/Replace File(file path (use dialog)=w286, error in=w290, operation (0:open)=T5."open or create") -> (refnum out=w296:refnum<file>, error out=w293:errorcluster)  [unwired: 3 in, 1 out]
            n99 = Write to Text File(file (use dialog)=w296, text=w295, error in=w293) -> (refnum out=w294:refnum<file>, error out=w292:errorcluster)  [unwired: 1 in, 1 out]
            n100 = Close File(refnum=w294, error in=w292) -> (path=w285:path, error out=w291:errorcluster)
            n101 = Bundle By Name(cluster=w288, "Self Reference"=w287, "Path"=w285) -> (w289:T7)
            n102 = call <vilib>:"Add State(s) to Queue__jki_lib_state_machine.vi"("State(s) in (\"\")"=w300) -> ("States Out"=w299:string)  [unwired: 14 in]
          }
          frame "Log: Close" {
            n103 = Unbundle By Name(w304) -> ("File Refnum"=w303:refnum<file>)
            n104 = Close File(refnum=w303, error in=w301) -> (error out=w302:errorcluster)  [unwired: 1 out]
            n105 = call <vilib>:"Add State(s) to Queue__jki_lib_state_machine.vi"("State(s) in (\"\")"=w307) -> ("States Out"=w306:string)  [unwired: 14 in]
          }
          frame "Log: Open" {
            n106 = Unbundle By Name(w308) -> ("Path"=w314:path)
            n107 = Open/Create/Replace File(file path (use dialog)=w314, error in=w311, operation (0:open)=T5."open") -> (refnum out=w310:refnum<file>, error out=w312:errorcluster)  [unwired: 3 in, 1 out]
            n108 = Bundle By Name(cluster=w308, "File Refnum"=w310) -> (w309:T7)
            n109 = call <vilib>:"Add State(s) to Queue__jki_lib_state_machine.vi"("State(s) in (\"\")"=w317) -> ("States Out"=w316:string)  [unwired: 14 in]
          }
          frame "Log: Append" {
            n110 = Unbundle By Name(w320) -> ("Active Log"=w326:string, "File Refnum"=w328:refnum<file>)
            n111 = Get File Size(file=w328, error in=w322) -> (refnum out=w329:refnum<file>, size (in bytes)=w330:i64, 0:w324:errorcluster)
            n112 = Set File Position(offset (in bytes) (0)=w330, refnum=w329, error in=w324) -> (refnum out=w327:refnum<file>, error out=w325:errorcluster)  [unwired: 1 out]
            n113 = Write to Text File(file (use dialog)=w327, text=w326, error in=w325) -> (refnum out=w319:refnum<file>, error out=w323:errorcluster)  [unwired: 1 in, 1 out]
            n114 = Bundle By Name(cluster=w320, "Active Log"="", "File Refnum"=w319) -> (w321:T7)
            n115 = call <vilib>:"Add State(s) to Queue__jki_lib_state_machine.vi"("State(s) in (\"\")"=w333) -> ("States Out"=w332:string)  [unwired: 14 in]
          }
          frame "Log: Path" {
            n116 = call "GenerateLogFilePath.vi"("error in (no error)"=w338) -> ("error out"=w337:errorcluster, "actual path"=w336:path)  [unwired: 9 in]
            n117 = Bundle By Name(cluster=w334, "Path"=w336) -> (w335:T7)
            n118 = call <vilib>:"Add State(s) to Queue__jki_lib_state_machine.vi"("State(s) in (\"\")"=w341) -> ("States Out"=w340:string)  [unwired: 14 in]
          }
        }
      }
    }
    frame Error {
    }
  }
  n119 = call-parent "Process.vi"("error in"=w7, "SMO"=w6) -> ("error out"=w4:errorcluster, "SMO out"=→"Log.Litho out":refnum<class "Log.Litho.lvclass">)  [unwired: 8 in]
  n120 = Merge Errors(w4, w3) -> (→"error out":errorcluster)
